vi "Set Scope Mode.vi"(8 "error in (no error)":errorcluster, 10 "Scope Mode (0: Off)":u32(ring) items=["Off", "AC & DC Voltage", "Edge", "Leveled Sine", "Marker", "Wave Generator", "Video", "Pulse", "Impedance & Capacitance Meas", "Overload"], 11 "VISA resource name":refnum<visa-resource-name>) -> (0 "error out":errorcluster {"code" format="%.0x"}, 3 "VISA resource name out":refnum<visa-resource-name>)   [LabVIEW 2013, in "Fluke 5XXX Series Multicalibrators.lvlib"]
doc: "This VI sets the oscilloscope’s mode of operation.\n\nOnce in SCOPE mode, use the FL5XMCAL Set Output Values.vi to program new output in all VIs except FL5XMCAL Impedance Measurement.vi and the FL5XMCAL Set Calibrator Range.vi as required (in OVERLD, PULSE, and MEAS Z functions only.)\n\nThe FL5XMCAL Get Function Type.vi returns the corresponding oscilloscope modes.\n\nNote:\n\nThis VI is available only for instrument models 5500A and 5520A with oscilloscope option SC300 (SC600 or SC1100)."
uses:
  Fluke 5XXX Series Multicalibrators.lvlib
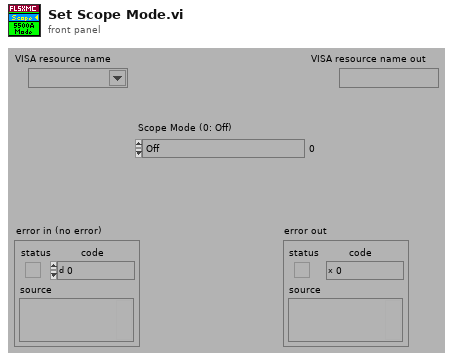
[diagram p1: front panel]
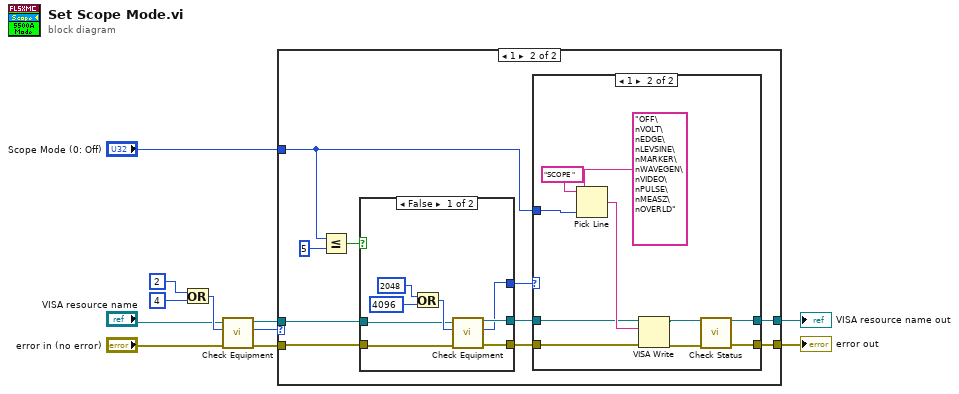
[diagram p0: block diagram]
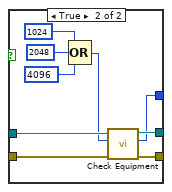
[diagram p4: hidden frame]
diagram:
  n1 = Or(x=2 ("Numeric"), y=4 ("Numeric")) -> (x .or. y?=w9:i32)
  n2 = call "Check Equipment.vi"("error in (no error)"="error in (no error)", "Bit Mask"=w9, "VISA resource name"="VISA resource name") -> ("error out"=w11:errorcluster, "Present?"=w1:u32, "VISA resource name out"=w10:refnum<visa-resource-name>)  [unwired: 6 in]
  n3 = case shown="1" w1 {
    tunnel: "Scope Mode (0: Off)" -> [_ w21]
    tunnel: [w12 w22] -> w3
    tunnel: w11 -> [w13 w18]
    tunnel: w10 -> [w12 w17]
    tunnel: [w13 w23] -> w2
    frame 0, Default {
    }
    frame 1 {
      n4 = Less Or Equal?(x=w21, y=u32 5) -> (x <= y?=w19:bool)
      n5 = case shown="False" w19 {
        tunnel: w18 -> [w38 w52]
        tunnel: w17 -> [w39 w51]
        tunnel: [w41 w50] -> w16
        tunnel: [w40 w49] -> w15
        tunnel: [w36 w44] -> w14
        frame False {
          n6 = Or(x=2048 ("Numeric"), y=4096 ("Numeric")) -> (x .or. y?=w43:i32)
          n7 = call "Check Equipment.vi"("error in (no error)"=w38, "Bit Mask"=w43, "VISA resource name"=w39) -> ("error out"=w41:errorcluster, "Present?"=w36:u32, "VISA resource name out"=w40:refnum<visa-resource-name>)  [unwired: 6 in]
        }
        frame True {
          n8 = Compound Arithmetic op=OR(1024 ("Numeric"), 2048 ("Numeric"), 4096 ("Numeric")) -> (w45:i32)
          n9 = call "Check Equipment.vi"("error in (no error)"=w52, "Bit Mask"=w45, "VISA resource name"=w51) -> ("error out"=w50:errorcluster, "Present?"=w44:u32, "VISA resource name out"=w49:refnum<visa-resource-name>)  [unwired: 6 in]
        }
      }
      n10 = case shown="1" w14 {
        tunnel: [w24 w26] -> w23
        tunnel: [w25 w30] -> w22
        tunnel: w21 -> [_ w29]
        tunnel: w16 -> [w24 w28]
        tunnel: w15 -> [w25 w27]
        frame 0, Default {
        }
        frame 1 {
          n11 = Pick Line(string ("")="SCOPE " ("Reset Command"), multi-line string="OFF\nVOLT\nEDGE\nLEVSINE\nMARKER\nWAVEGEN\nVIDEO\nPULSE\nMEASZ\nOVERLD", line index=w29) -> (output string=w33:string)
          n12 = VISA Write(VISA resource name=w27, write buffer=w33, error in (no error)=w28) -> (VISA resource name out=w31:refnum<visa-resource-name>, error out=w32:errorcluster)  [unwired: 1 out]
          n13 = call "Check Status.vi"("VISA resource name"=w31, "error in (no error)"=w32) -> ("VISA resource name out"=w30:refnum<visa-resource-name>, "error out"=w26:errorcluster)  [unwired: 12 in]
        }
      }
    }
  }
  "VISA resource name out" <- w3
  "error out" <- w2
